vi "isSim.vi"(8 "error in (no error)":errorcluster, 11 "TecellaClient in":refnum<class "TecellaClient.lvclass">) -> (0 "error out":errorcluster, 2 "Is Simulated?":bool, 3 "TecellaClient out":refnum<class "TecellaClient.lvclass">)   [LabVIEW 2009, in "TecellaClient.lvclass"]
uses:
  TecellaClient.lvclass
panel:
  out "Data Returned":string
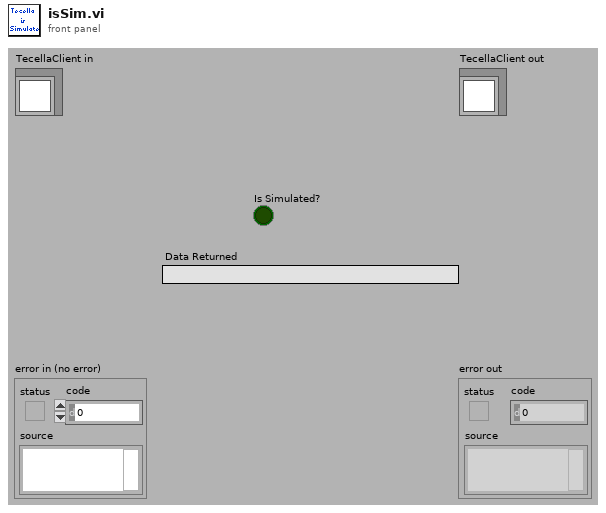
[diagram p1: front panel]
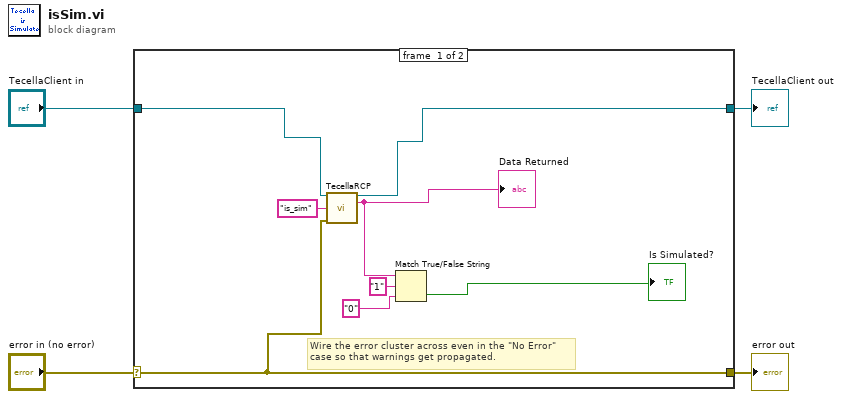
[diagram p0: block diagram]
diagram:
  n1 = case shown="No Error" "error in (no error)" {
    selector: "error in (no error)" -> [w6 w14]
    tunnel: [w6 w14] -> w3
    tunnel: [w7 w13] -> w1
    tunnel: "TecellaClient in" -> [w8 w13]
    frame #0 {
      # "Wire the error cluster across even in the \"No Error\"\ncase so that warnings get propagated."
      n2 = call-dynamic "TecellaRCP.vi"("TecellaClient in"=w8, "method"="is_sim", "error in (no error)"=w6) -> ("TecellaClient out"=w7:refnum<class "TecellaClient.lvclass">, "Data Returned"=w10:string)  [unwired: 10 in, 1 out]
      "Data Returned" <- w10
      n3 = Match True/False String(2:"0" ("false string"), 3:"1" ("true string"), 4:w10) -> (0:→"Is Simulated?":bool)  [unwired: 1 out]
    }
    frame #1 {
    }
  }
  "error out" <- w3
  "TecellaClient out" <- w1
